vi "TempAverager.vi"(11 "Array in":dbl[](array[numeric])) -> (3 "Array out":dbl[](array[numeric]))   [LabVIEW 2018, in "Inputs.lvlib"]
uses:
  Inputs.lvlib
  <vilib>/ptbypt/NI_PtbyPt.lvlib
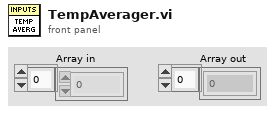
[diagram p1: front panel]
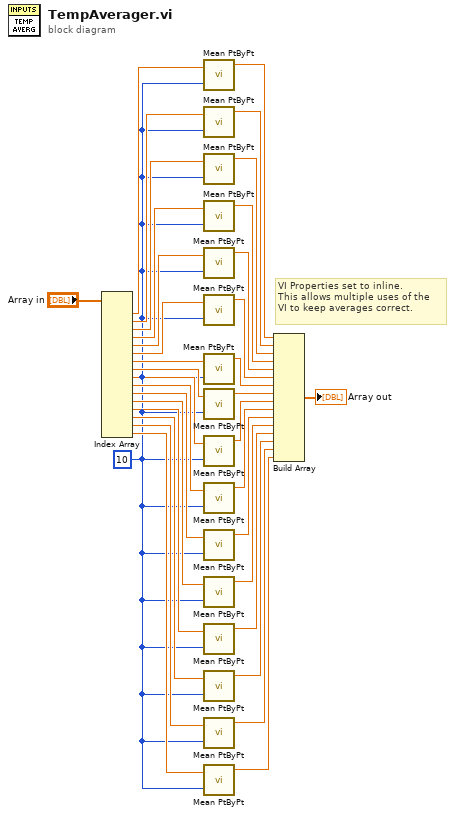
[diagram p0: block diagram]
diagram:
  w3 = 10 ("sample length")
  # "VI Properties set to inline. \nThis allows multiple uses of the \nVI to keep averages correct."
  n1 = Index Array(array="Array in") -> (element #1=w20:dbl, element #2=w21:dbl, element #3=w22:dbl, element #4=w23:dbl, element #5=w24:dbl, element #6=w25:dbl, element #7=w26:dbl, element #8=w27:dbl, element #9=w28:dbl, element #10=w29:dbl, element #11=w30:dbl, element #12=w31:dbl, element #13=w32:dbl, element #14=w33:dbl, element #15=w34:dbl, element #16=w35:dbl)  [unwired: 16 in]
  n2 = call <vilib>:"Mean PtByPt.vi"("x"=w20, "sample length"=w3) -> ("mean"=w2:dbl)  [unwired: 2 in, 1 out]
  n3 = call <vilib>:"Mean PtByPt.vi"("x"=w21, "sample length"=w3) -> ("mean"=w4:dbl)  [unwired: 2 in, 1 out]
  n4 = call <vilib>:"Mean PtByPt.vi"("x"=w22, "sample length"=w3) -> ("mean"=w5:dbl)  [unwired: 2 in, 1 out]
  n5 = call <vilib>:"Mean PtByPt.vi"("x"=w23, "sample length"=w3) -> ("mean"=w6:dbl)  [unwired: 2 in, 1 out]
  n6 = call <vilib>:"Mean PtByPt.vi"("x"=w24, "sample length"=w3) -> ("mean"=w7:dbl)  [unwired: 2 in, 1 out]
  n7 = call <vilib>:"Mean PtByPt.vi"("x"=w25, "sample length"=w3) -> ("mean"=w8:dbl)  [unwired: 2 in, 1 out]
  n8 = call <vilib>:"Mean PtByPt.vi"("x"=w26, "sample length"=w3) -> ("mean"=w9:dbl)  [unwired: 2 in, 1 out]
  n9 = call <vilib>:"Mean PtByPt.vi"("x"=w27, "sample length"=w3) -> ("mean"=w10:dbl)  [unwired: 2 in, 1 out]
  n10 = call <vilib>:"Mean PtByPt.vi"("x"=w28, "sample length"=w3) -> ("mean"=w11:dbl)  [unwired: 2 in, 1 out]
  n11 = call <vilib>:"Mean PtByPt.vi"("x"=w29, "sample length"=w3) -> ("mean"=w12:dbl)  [unwired: 2 in, 1 out]
  n12 = call <vilib>:"Mean PtByPt.vi"("x"=w30, "sample length"=w3) -> ("mean"=w13:dbl)  [unwired: 2 in, 1 out]
  n13 = call <vilib>:"Mean PtByPt.vi"("x"=w31, "sample length"=w3) -> ("mean"=w14:dbl)  [unwired: 2 in, 1 out]
  n14 = call <vilib>:"Mean PtByPt.vi"("x"=w32, "sample length"=w3) -> ("mean"=w15:dbl)  [unwired: 2 in, 1 out]
  n15 = call <vilib>:"Mean PtByPt.vi"("x"=w33, "sample length"=w3) -> ("mean"=w16:dbl)  [unwired: 2 in, 1 out]
  n16 = call <vilib>:"Mean PtByPt.vi"("x"=w34, "sample length"=w3) -> ("mean"=w17:dbl)  [unwired: 2 in, 1 out]
  n17 = call <vilib>:"Mean PtByPt.vi"("x"=w35, "sample length"=w3) -> ("mean"=w18:dbl)  [unwired: 2 in, 1 out]
  n18 = Build Array(w2, w4, w5, w6, w7, w8, w9, w10, w11, w12, w13, w14, w15, w16, w17, w18) -> (→"Array out":dbl[])
